vi "prescanHoldTime.vi"(8 "error in (no error)":errorcluster, 11 "GuassianNoiseWave in":refnum<class "GuassianNoiseWave.lvclass">) -> (0 "error out":errorcluster, 2 "PrescanHold?":bool=TRUE, 3 "GuassianNoiseWave out":refnum<class "GuassianNoiseWave.lvclass">)   [LabVIEW 2015, in "GuassianNoiseWave.lvclass"]
uses:
  GuassianNoiseWave.lvclass
  GuassianNoiseWave.lvclass/GuassianNoiseWave.ctl
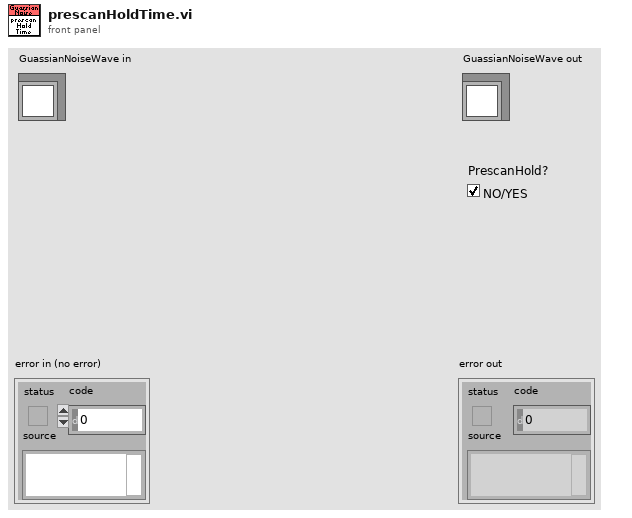
[diagram p1: front panel]
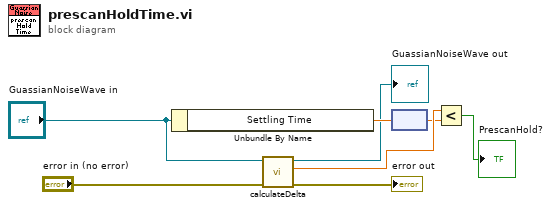
[diagram p0: block diagram]
diagram:
  n1 = Unbundle By Name("GuassianNoiseWave in") -> ("Settling Time"=w7:dbl[unit])
  n2 = call "calculateDelta.vi"("error in (no error)"="error in (no error)", "GuassianNoiseWave in"="GuassianNoiseWave in") -> ("error out"=→"error out":errorcluster, "Delta Timestamp"=w6:dbl, "GuassianNoiseWave out"=→"GuassianNoiseWave out":refnum<class "GuassianNoiseWave.lvclass">)  [unwired: 7 in]
  n3 = node(w7) -> (w5:dbl)
  n4 = Less?(x=w6, y=w5) -> (x < y?=→"PrescanHold?":bool)
